vi "Aula4.vi"() -> ()   [LabVIEW 2024]
uses:
  <vilib>/numeric/Random Number (Range) DBL.vi
panel:
  out "Pontência ativa fase C 3":dbl[](graph)
  out "Pontência ativa fase B 2":dbl[](graph)
  out "Potência Ativa C 3":dbl[](array[numeric])
  out "Corrente C3":dbl[](array[numeric])
  out "Tensão C 3":dbl[](array[numeric])
  out "Potência Ativa B 2":dbl[](array[numeric])
  out "Corrente B 2":dbl[](array[numeric])
  out "Tensão B 2":dbl[](array[numeric])
  out "Potência Ativa A":dbl[](array[numeric])
  out "Corrente A":dbl[](array[numeric])
  out "Tensão A":dbl[](array[numeric])
  out "Fator de potência":dbl
  in  "Limite superior FP":dbl=100.0
  in  "Limite inferior FP":dbl
  out "Pontência ativa fase A":dbl[](graph)
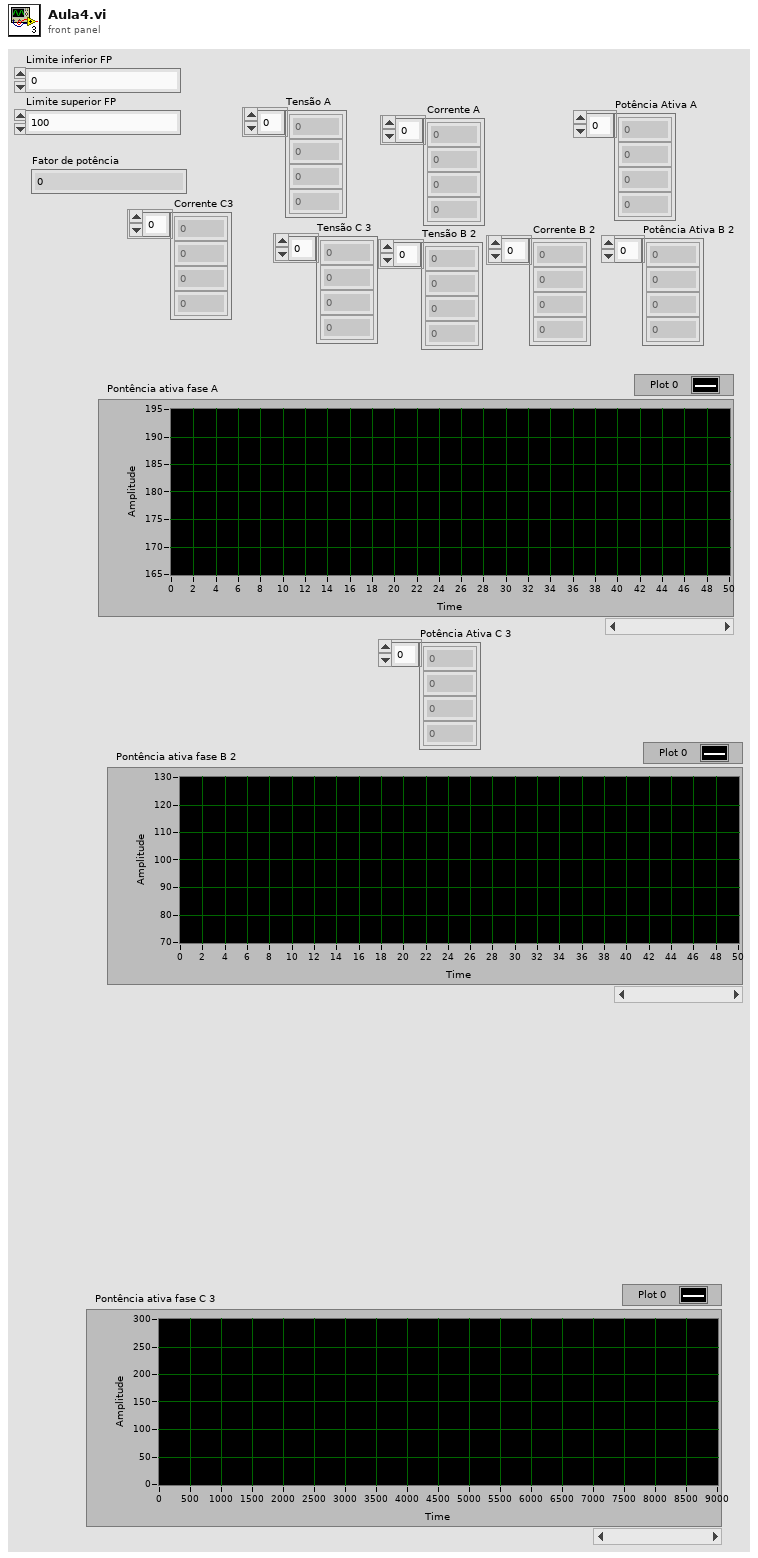
[diagram p1: front panel]
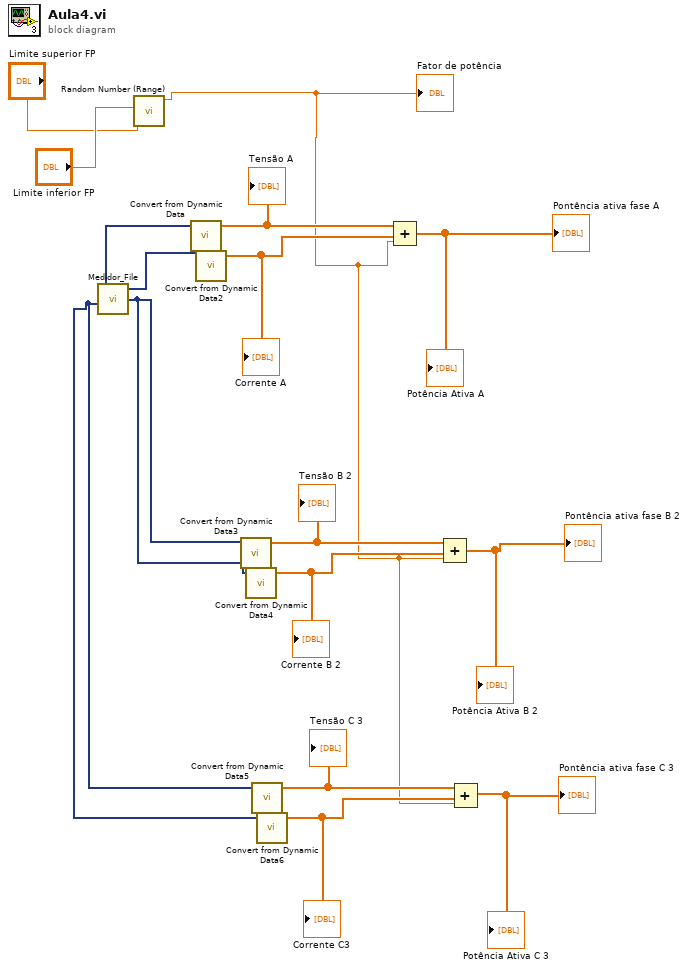
[diagram p0: block diagram]
diagram:
  n1 = call "Medidor_File.vi"() -> ("Corrente Fase B"=w4:dynamicdata, "Corrente Fase A"=w16:dynamicdata, "Tensão Fase C"=w3:dynamicdata, "Tensão Fase A"=w15:dynamicdata)  [unwired: 3 out]
  n2 = call-poly <vilib>:"Random Number (Range).vi"("lower bound (0)"="Limite inferior FP", "upper bound (100)"="Limite superior FP") -> ("number"=w5:dbl)  [unwired: 9 in]
  "Fator de potência" <- w5
  n3 = call "Convert from Dynamic Data"("Dynamic Data Type"=w15) -> ("Array"=w14:dbl[])  [unwired: 3 in]
  "Tensão A" <- w14
  n4 = call "Convert from Dynamic Data2"("Dynamic Data Type"=w16) -> ("Array"=w13:dbl[])  [unwired: 3 in]
  "Corrente A" <- w13
  n5 = call "Convert from Dynamic Data3"("Dynamic Data Type"=w4) -> ("Array"=w9:dbl[])  [unwired: 3 in]
  "Tensão B 2" <- w9
  n6 = call "Convert from Dynamic Data4"("Dynamic Data Type"=w4) -> ("Array"=w8:dbl[])  [unwired: 3 in]
  "Corrente B 2" <- w8
  n7 = call "Convert from Dynamic Data5"("Dynamic Data Type"=w3) -> ("Array"=w7:dbl[])  [unwired: 3 in]
  "Tensão C 3" <- w7
  n8 = call "Convert from Dynamic Data6"("Dynamic Data Type"=w3) -> ("Array"=w6:dbl[])  [unwired: 3 in]
  "Corrente C3" <- w6
  n9 = Compound Arithmetic op=ADD(w14, w13, w5) -> (→"Pontência ativa fase A" →"Potência Ativa A":dbl[])
  n10 = Compound Arithmetic op=ADD(w9, w8, w5) -> (→"Potência Ativa B 2" →"Pontência ativa fase B 2":dbl[])
  n11 = Compound Arithmetic op=ADD(w7, w6, w5) -> (→"Potência Ativa C 3" →"Pontência ativa fase C 3":dbl[])
